vi "ConfigurePIDs.vi"(8 "error in (no error)":errorcluster, 11 "connection info":T1) -> (0 "error out":errorcluster, 3 "connection info":T1)   [LabVIEW 2015, in "Diagnostics Host Automation API.lvlib"]
uses:
  Diagnostics Host Automation API.lvlib
  <vilib>/NI/STM/TCP/TCP Connection Info.ctl
  <vilib>/NI/STM/SubVIs/MetaDataElement.ctl
  <vilib>/NI/STM/TCP/Write Message (TCP).vi
  <vilib>/NI/STM/NI STM.lvlib
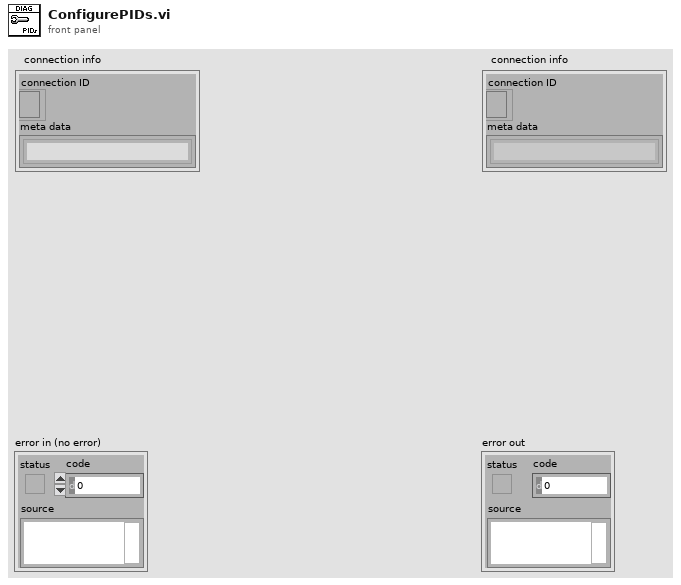
[diagram p1: front panel]
types:
  T1 = typedef "NI STM.lvlib/TCP Connection Info.ctl" = cluster{"connection ID":refnum<k5>, "meta data":T2[]}
  T2 = typedef "NI STM.lvlib/MetaDataElement.ctl" = string
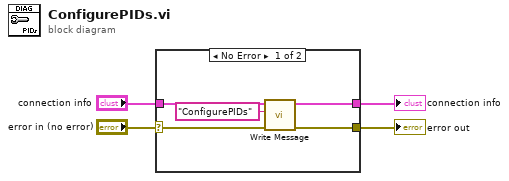
[diagram p0: block diagram]
diagram:
  n1 = case shown="No Error" "error in (no error)" {
    selector: "error in (no error)" -> [w5 w11]
    tunnel: "connection info" -> [w9 w10]
    tunnel: [w8 w10] -> w3
    tunnel: [w7 w11] -> w2
    frame No Error {
      n2 = call-poly <vilib>:"Write Message.vi"("error in"=w5, "name"="ConfigurePIDs" ("Name"), "connection info in"=w9) -> ("error out"=w7:errorcluster, "connection info out"=w8:T1)  [unwired: 7 in]
    }
    frame Error {
    }
  }
  "connection info" <- w3
  "error out" <- w2
